vi "getAvarageVoltageForInterval.vi"(7 "interval(sec)":dbl, 8 "lastVal":dbl format="%.6f", 10 "voltages":dbl[](array[numeric]) format="%.6f", 11 "timeArray":dbl[](array[numeric]) format="%<%H:%M:%S>t") -> (3 "avarage":dbl format="%.6f")   [LabVIEW 2018]
panel:
  out "x-y":dbl[](array[numeric])
  out "elements":dbl
  out "idx":i32
  out "deleted portion":dbl[](array[numeric]) format="%.6f"
  out "min value":dbl format="%<%H:%M:%S>t"
  out "max value":dbl format="%<%H:%M:%S>t"
  out "timeDiff":dbl format="%<%H:%M:%S>t"
  out "last":dbl format="%<%H:%M:%S>t"
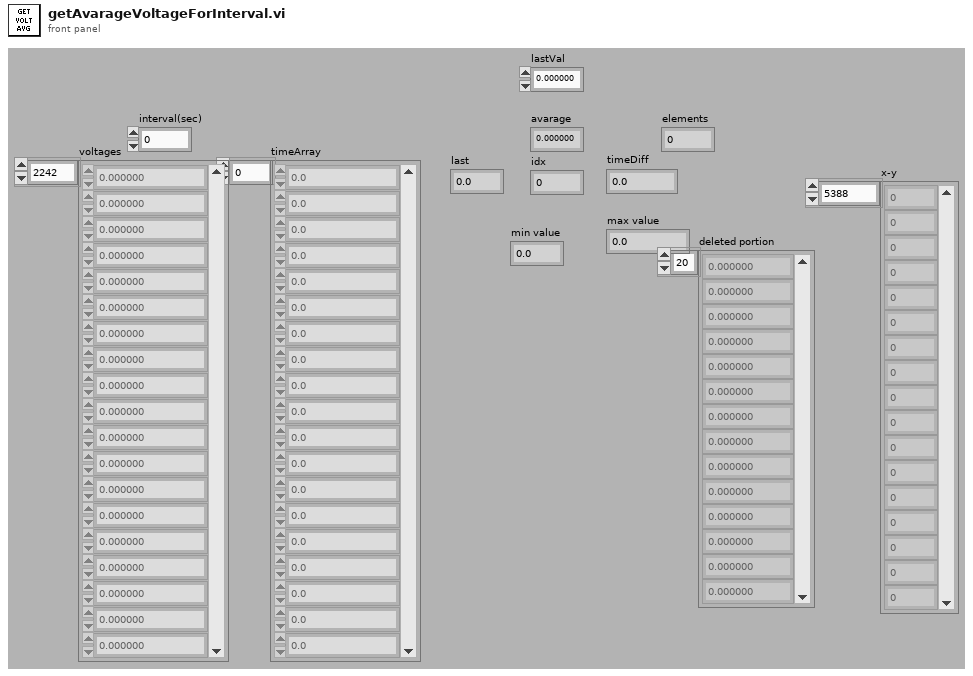
[diagram p1: front panel]
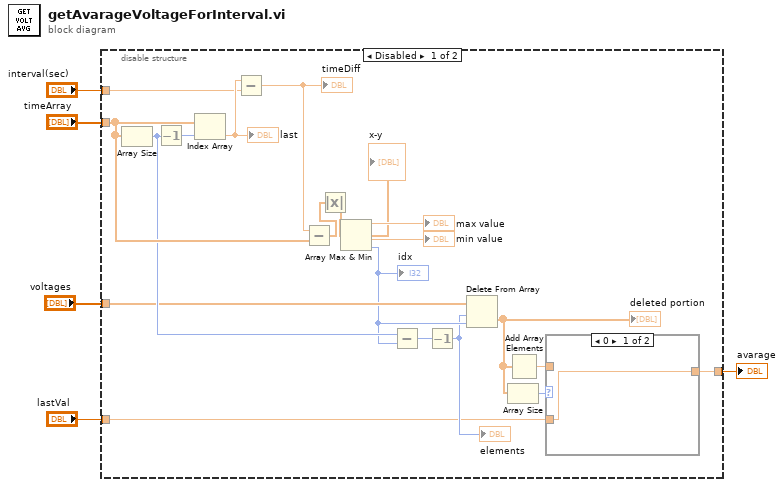
[diagram p0: block diagram]
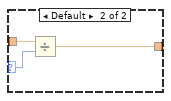
[diagram p2: hidden frame]
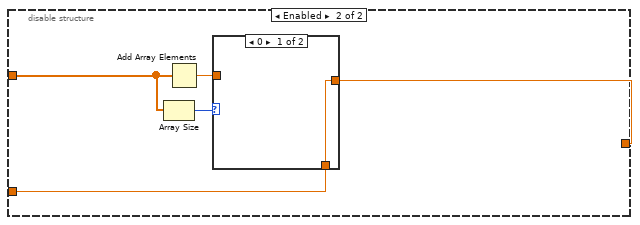
[diagram p3: hidden frame]
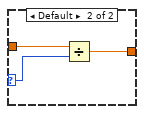
[diagram p4: hidden frame]
diagram:
  n1 = disable-structure shown="Disabled" {
    disable-tunnel: "timeArray" -> [w19 _]
    disable-tunnel: "interval(sec)" -> [w15 _]
    disable-tunnel: "voltages" -> [w12 w33]
    disable-tunnel: [w9 w30] -> w2
    disable-tunnel: "lastVal" -> [w8 w29]
    frame Disabled {
      n2 = Array Size(array=w19) -> (size(s)=w18:i32)
      n3 = Decrement(x=w18) -> (x-1=w23:i32)
      n4 = Index Array(array=w19, index=w23) -> (element=w24:dbl)
      "last" <- w24
      n5 = Subtract(x=w24, y=w15) -> (x-y=w22:dbl)
      "timeDiff" <- w22
      n6 = Subtract(x=w22, y=w19) -> (x-y=w14:dbl[])
      n7 = Absolute Value(x=w14) -> (abs(x)=w13:dbl[])
      "x-y" <- w13
      n8 = Array Max & Min(array=w13) -> (max value=→"max value":dbl, min value=→"min value":dbl, min index (indices)=w11:i32)  [unwired: 1 out]
      "idx" <- w11
      n9 = Subtract(x=w18, y=w11) -> (x-y=w20:i32)
      n10 = Decrement(x=w20) -> (x-1=w10:i32)
      "elements" <- w10
      n11 = Delete From Array(array=w12, length=w10, index=w11) -> (deleted portion=w7:dbl[])  [unwired: 1 out]
      "deleted portion" <- w7
      n12 = Array Size(array=w7) -> (size(s)=w6:i32)
      n13 = Add Array Elements(numeric array=w7) -> (sum=w16:dbl)
      n14 = case shown="0" w6 {
        selector: w6 -> [_ w26]
        tunnel: w16 -> [_ w28]
        tunnel: [w25 w27] -> w9
        tunnel: w8 -> [w25 _]
        frame 0 {
        }
        frame Default {
          n15 = Divide(x=w28, y=w26) -> (x/y=w27:dbl)
        }
      }
    }
    frame Enabled {
      n16 = Array Size(array=w33) -> (size(s)=w32:i32)
      n17 = Add Array Elements(numeric array=w33) -> (sum=w31:dbl)
      n18 = case shown="0" w32 {
        selector: w32 -> [_ w36]
        tunnel: w31 -> [_ w37]
        tunnel: [w34 w35] -> w30
        tunnel: w29 -> [w34 _]
        frame 0 {
        }
        frame Default {
          n19 = Divide(x=w37, y=w36) -> (x/y=w35:dbl)
        }
      }
    }
  }
  "avarage" <- w2
